vi "ProgramFreqBulk.vi"(8 "error in (no error)":errorcluster, 9 "auto start":bool=TRUE, 11 "RUS settings":T1={"NI-DAQ lockin settings"={"Samples per sine wave"=0, "Sine waves per freq step"=0, "Output Representation"=enum."Real/Imaginary", "Low-pass filter"=enum."Butterworth", "Ranges and couplings "=[]}, "Fast swep settings"={"Update rate (Hz)"=250.0, "Start F, Hz"=200000.0, "Stop F"=1700000.0, "Number of points"=30000, "Amplitude"=2.1, "Init&amplitude"=TRUE, "IF"=1000.0, "Time constant"=0.1}, "Pre-sweep delay, s"=0.0, "Lockin mode"=enum."NI-DAQ", "SR Lockin"="GPIB0::10::INSTR", "DAQmx Device"="Dev3", "Clock Multiplier"=64, "Fast Sweep Data Out"={"DO clock task"="", "DO task"="", "Update clock task"="", "DAQ lockin task"="", "Pre-sweep counter task"=""}, "Lockin Range, V"=0.0, "F Array"=[], "Freq. update clock terminal"="", "DO Clock Rate (Hz)"=5000000.0, "ADC clock terminal"="/PFI4", "Pre-sweep counter terminal"="", "Samples per read"=10, "DO clock terminal"="", "Pre-sweep points"=0, "F points per write"=1000, "Total sweep time, s"=0.0, "Initial SYNTH phase"=0.0, "Record IF"=FALSE, "Save data settings"={"Save data"=TRUE, "Data Root Path"=path "", "File Prefix"="", "File Format"=enum."ASCII", "Save column names"=TRUE, "File Comments"="<Description of the current file>", "User/Prj"="<User Name/Project Description>"}, "Data file path"=path "", "New data user event"=refnum, "Stop user event"=refnum, "Number of channels"=1, "Auto-phase"=FALSE, "RP Transeiver"=refnum} {"Lockin Range, V" format="%#_6e"; "Fast swep settings"."IF" format="%#_6p"; "Fast swep settings"."Amplitude" min=0.0 max=2.5; "Fast swep settings"."Number of points" format="%.0p"; "Fast swep settings"."Stop F" format="%#_6p"; "Fast swep settings"."Start F, Hz" format="%#_6p"; "Fast swep settings"."Update rate (Hz)" format="%0.2f"; "NI-DAQ lockin settings"."Ranges and couplings"."Coupling" items=["default"=-1, "RSE"=10083, "NRSE"=10078, "Differential"=10106, "Pseudodifferential"=12529]}) -> (0 "error out":errorcluster, 2 "SpaceAvail":u32, 3 "RUS settings out":T1={"NI-DAQ lockin settings"={"Samples per sine wave"=0, "Sine waves per freq step"=0, "Output Representation"=enum."Real/Imaginary", "Low-pass filter"=enum."Butterworth", "Ranges and couplings "=[]}, "Fast swep settings"={"Update rate (Hz)"=250.0, "Start F, Hz"=200000.0, "Stop F"=1700000.0, "Number of points"=30000, "Amplitude"=2.1, "Init&amplitude"=TRUE, "IF"=1000.0, "Time constant"=0.1}, "Pre-sweep delay, s"=0.0, "Lockin mode"=enum."NI-DAQ", "SR Lockin"="GPIB0::10::INSTR", "DAQmx Device"="Dev3", "Clock Multiplier"=64, "Fast Sweep Data Out"={"DO clock task"="", "DO task"="", "Update clock task"="", "DAQ lockin task"="", "Pre-sweep counter task"=""}, "Lockin Range, V"=0.0, "F Array"=[], "Freq. update clock terminal"="", "DO Clock Rate (Hz)"=5000000.0, "ADC clock terminal"="/PFI4", "Pre-sweep counter terminal"="", "Samples per read"=10, "DO clock terminal"="", "Pre-sweep points"=0, "F points per write"=1000, "Total sweep time, s"=0.0, "Initial SYNTH phase"=0.0, "Record IF"=FALSE, "Save data settings"={"Save data"=TRUE, "Data Root Path"=path "", "File Prefix"="", "File Format"=enum."ASCII", "Save column names"=TRUE, "File Comments"="<Description of the current file>", "User/Prj"="<User Name/Project Description>"}, "Data file path"=path "", "New data user event"=refnum, "Stop user event"=refnum, "Number of channels"=1, "Auto-phase"=FALSE, "RP Transeiver"=refnum} {"Lockin Range, V" format="%#_6e"; "Fast swep settings"."IF" format="%#_6p"; "Fast swep settings"."Amplitude" min=0.0 max=2.5; "Fast swep settings"."Number of points" format="%.0p"; "Fast swep settings"."Stop F" format="%#_6p"; "Fast swep settings"."Start F, Hz" format="%#_6p"; "Fast swep settings"."Update rate (Hz)" format="%0.2f"; "NI-DAQ lockin settings"."Ranges and couplings"."Coupling" items=["default"=-1, "RSE"=10083, "NRSE"=10078, "Differential"=10106, "Pseudodifferential"=12529]}, 4 "DO array  making time":u32, 6 "DO write time":u32)   [LabVIEW 2015]
uses:
  RUS/Controls/RUS settings.ctl
  NHMFL_Core/Libraries/Red Pitaya/RP Core/RP Transceiver/RP Transceiver.lvclass
  RUS/Controls/RUS NI-DAQ Lockin Settings.ctl
  RUS/Controls/Sweep settings.ctl
  RUS/Controls/Lockin mode.ctl
  NHMFL_Core/Libraries/File/Controls/Save data settings.ctl
  NHMFL_Core/Libraries/File/Controls/File formats.ctl
  <vilib>/DAQmx/write.llb/DAQmx Write (Digital 1D U8 1Chan NSamp).vi
  <vilib>/DAQmx/miscellaneous.llb/DAQmx Fill In Error Info.vi
  <resource>/objmgr/daqmx.rc
panel:
  in  "auto start 2":bool=TRUE
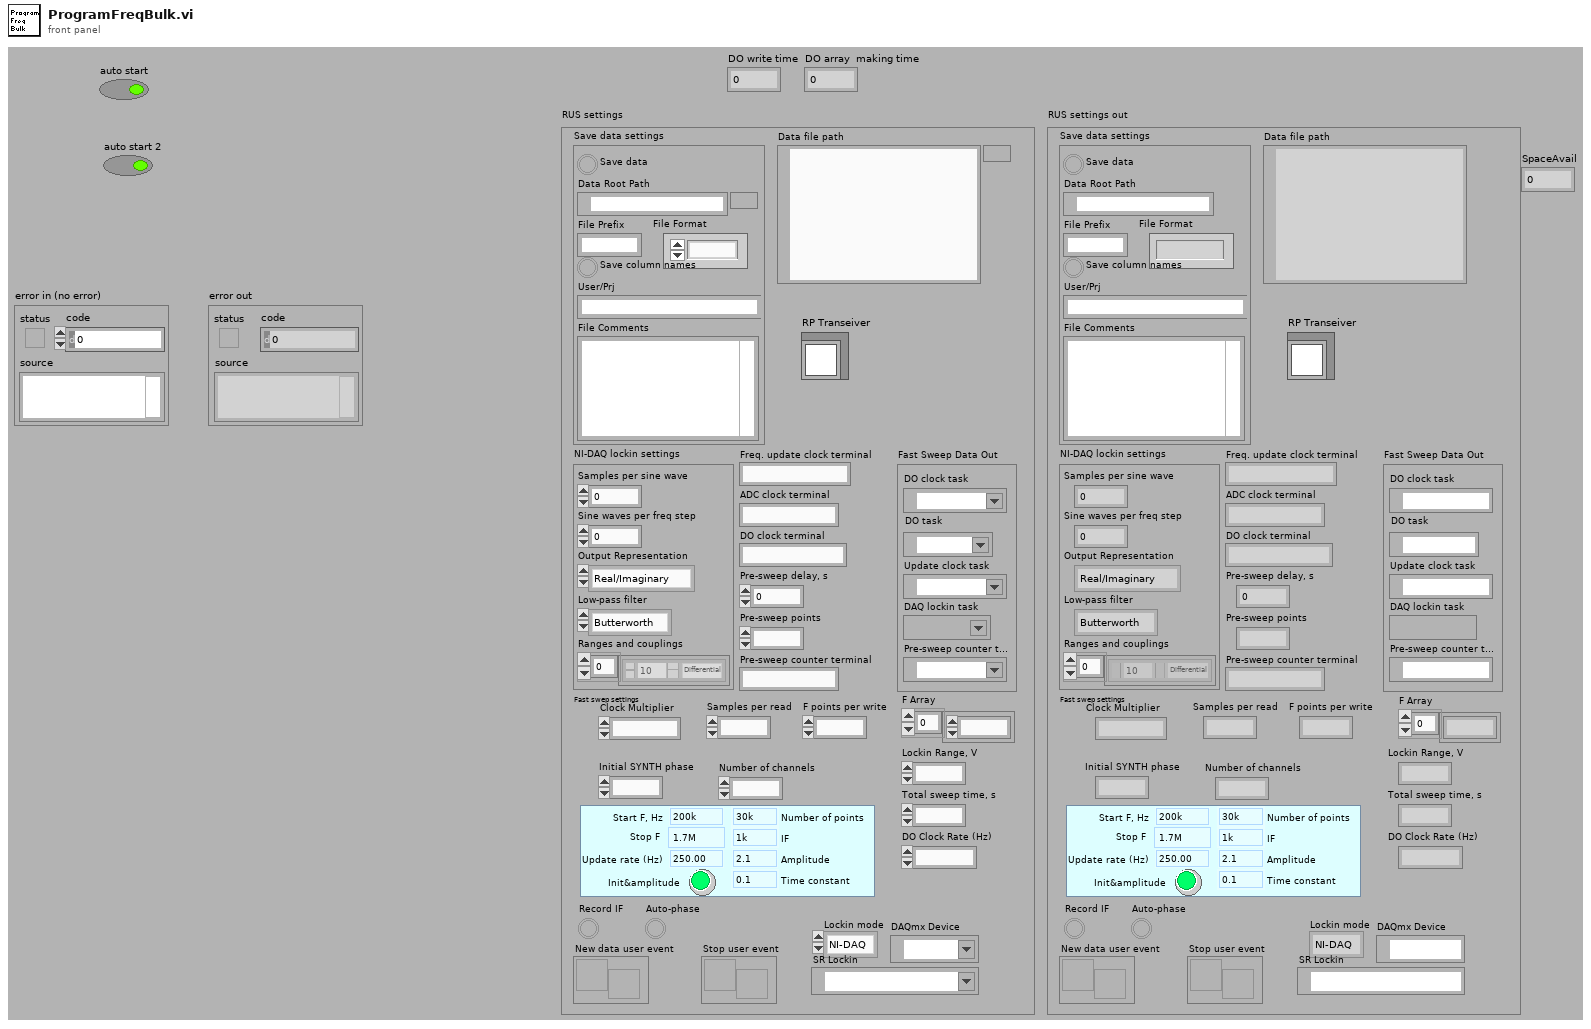
[diagram p1: front panel]
types:
  T1 = typedef "RUS settings.ctl" = cluster{"NI-DAQ lockin settings":T2, "Fast swep settings":T3, "Pre-sweep delay, s":dbl, "Lockin mode":T4, "SR Lockin":refnum<visa-resource-name>, "DAQmx Device":tag, "Clock Multiplier":i32, "Fast Sweep Data Out":cluster{"DO clock task":refnum<k21>, "DO task":refnum<k21>, "Update clock task":refnum<k21>, "DAQ lockin task":refnum<k21>, "Pre-sweep counter task":refnum<k21>}, "Lockin Range, V":sgl, "F Array":dbl[], "Freq. update clock terminal":string, "DO Clock Rate (Hz)":dbl, "ADC clock terminal":string, "Pre-sweep counter terminal":string, "Samples per read":i32, "DO clock terminal":string, "Pre-sweep points":i32, "F points per write":i32, "Total sweep time, s":dbl, "Initial SYNTH phase":dbl, "Record IF":bool, "Save data settings":T5, "Data file path":path, "New data user event":refnum<user-event>, "Stop user event":refnum<user-event>, "Number of channels":i32, "Auto-phase":bool, "RP Transeiver":refnum<class "RP Transceiver.lvclass">}
  T2 = typedef "RUS NI-DAQ Lockin Settings.ctl" = cluster{"Samples per sine wave":i32, "Sine waves per freq step":i32, "Output Representation":enum16{"Real/Imaginary", "Polar"}, "Low-pass filter":enum16{"No filtering", "Butterworth", "Bessel"}, "Ranges and couplings ":cluster{"Range":dbl, "Coupling":i32}[]}
  T3 = typedef "Sweep settings.ctl" = cluster{"Update rate (Hz)":dbl, "Start F, Hz":dbl, "Stop F":dbl, "Number of points":i32, "Amplitude":dbl, "Init&amplitude":bool, "IF":dbl, "Time constant":dbl}
  T4 = typedef "Lockin mode.ctl" = enum16{"SRS", "NI-DAQ", "Pitaya"}
  T5 = typedef "Save data settings.ctl" = cluster{"Save data":bool, "Data Root Path":path, "File Prefix":string, "File Format":T6, "Save column names":bool, "File Comments":string, "User/Prj":string}
  T6 = typedef "File formats.ctl" = enum16{"TDMS", "ASCII", "BINARY"}
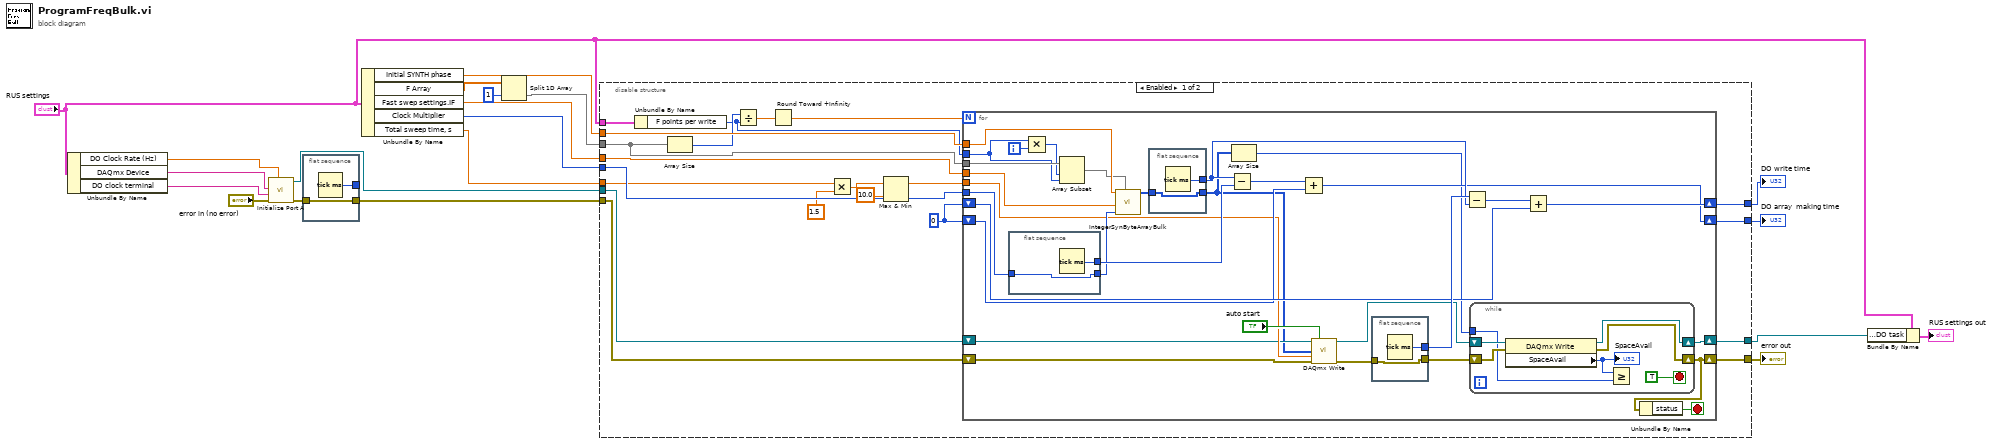
[diagram p0: block diagram]
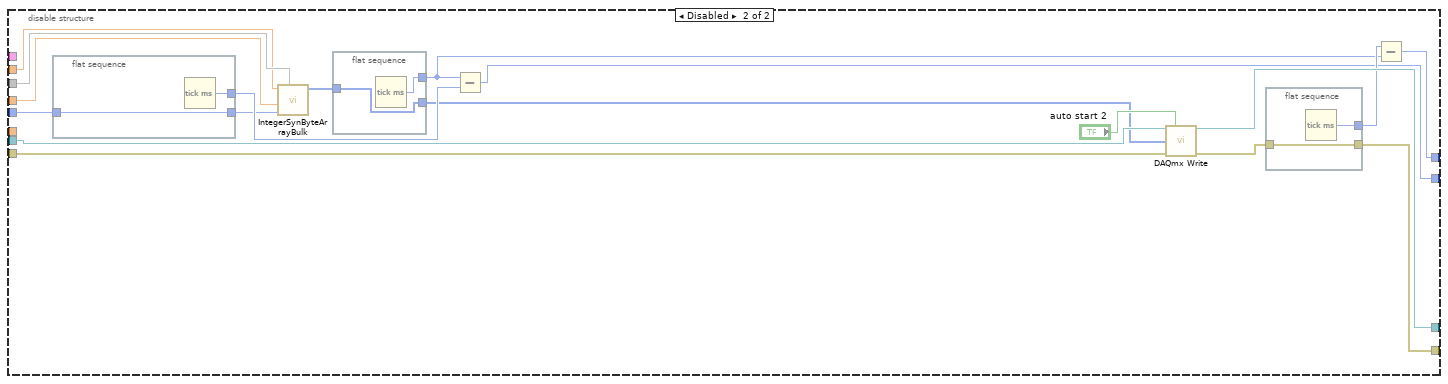
[diagram p2: hidden frame]
diagram:
  n1 = Unbundle By Name("RUS settings") -> ("DO Clock Rate (Hz)"=w14:dbl, "DAQmx Device"=w15:tag, "DO clock terminal"=w16:string)
  n2 = call "Initialize Port A.VI"("DO Clock Rate (Hz)"=w14, "error in (no error)"="error in (no error)", "Clock source"=w16, "DAQmx Device Name"=w15) -> ("error out"=w11:errorcluster, "task out"=w19:refnum<k21>)  [unwired: 3 in, 3 out]
  n3 = flat-sequence {
    tunnel: [w22] -> w10
    tunnel: w11 -> [w22]
    tunnel: [w21] -> _
    frame #0 {
      n4 = Tick Count (ms)() -> (millisecond timer value=w21:u32)
    }
  }
  n5 = Unbundle By Name("RUS settings") -> ("Initial SYNTH phase"=w3:dbl, "F Array"=w7:dbl[], "Fast swep settings.IF"=w6:dbl, "Clock Multiplier"=w13:i32, "Total sweep time, s"=w4:dbl)
  n6 = Split 1D Array(array=w7, index=1) -> (second subarray=w2:dbl[])  [unwired: 1 out]
  n7 = disable-structure shown="Enabled" {
    disable-tunnel: w19 -> [w25 w104]
    disable-tunnel: [w43 w103] -> w17
    disable-tunnel: w13 -> [w42 w102]
    disable-tunnel: [w41 w100] -> w12
    disable-tunnel: w10 -> [w24 w99]
    disable-tunnel: [w40 w97] -> w9
    disable-tunnel: [w39 w95] -> w8
    disable-tunnel: w2 -> [w37 w94]
    disable-tunnel: w3 -> [w38 w93]
    disable-tunnel: w6 -> [w33 w92]
    disable-tunnel: "RUS settings" -> [w27 _]
    disable-tunnel: w4 -> [w23 _]
    frame Enabled {
      w34 = u32 0
      n8 = Unbundle By Name(w27) -> ("F points per write"=w26:i32)
      n9 = Array Size(array=w37) -> (size(s)=w32:i32)
      n10 = Divide(x=w32, y=w26) -> (x/y=w36:dbl)
      n11 = Round Toward +Infinity(x=w36) -> (ceil(x): smallest int >= x=w35:dbl)
      n12 = Multiply(x=w23, y=1.5) -> (x*y=w29:dbl)
      n13 = Max & Min(x=w29, y=10.0) -> (max(x,y)=w30:dbl)  [unwired: 1 out]
      n14 = for {
        N: w35 -> [_]
        tunnel: w42 -> [w73]
        tunnel: w37 -> [w62]
        tunnel: w38 -> [w67]
        tunnel: w33 -> [w66]
        shift-right: [w45] -> w41
        shift-left: w24 -> [w52]
        shift-right: [w48] -> w43
        shift-left: w25 -> [w49]
        shift-right: [w60] -> w40
        shift-left: w34 -> [w59]
        shift-right: [w58] -> w39
        shift-left: w34 -> [w57]
        tunnel: w26 -> [w55]
        tunnel: w30 -> [w53]
        i -> [w56]
        stop <- w44 stop-if-true
        n15 = flat-sequence {
          tunnel: [w87] -> w65
          tunnel: w73 -> [w87]
          tunnel: [w86] -> w69
          frame #0 {
            n16 = Tick Count (ms)() -> (millisecond timer value=w86:u32)
          }
        }
        n17 = Multiply(x=w55, y=w56) -> (x*y=w54:i32)
        n18 = Array Subset(array=w62, index=w54, length=w55) -> (w61:dbl[])
        n19 = call "IntegerSynByteArrayBulk.vi"("Input  F1 array"=w61, "Clock multiplier"=w65, "Local Oscillator (IF,f2)"=w66, "Phase (degrees)"=w67) -> ("output array"=w64:u8[])  [unwired: 7 in]
        n20 = flat-sequence {
          tunnel: [w83] -> w47
          tunnel: w64 -> [w83]
          tunnel: [w82] -> w63
          frame #0 {
            n21 = Tick Count (ms)() -> (millisecond timer value=w82:u32)
          }
        }
        n22 = Subtract(x=w63, y=w69) -> (x-y=w68:u32)
        n23 = Array Size(array=w47) -> (size(s)=w46:i32)
        n24 = Add(x=w68, y=w57) -> (x+y=w58:u32)
        n25 = call-poly <vilib>:"DAQmx Write.vi"("task/channels in"=w49, "auto start"="auto start", "data"=w47, "timeout"=w53, "error in"=w52) -> ("task out"=w50:refnum<k21>, "error out"=w72:errorcluster)  [unwired: 9 out]
        n26 = flat-sequence {
          tunnel: [w85] -> w51
          tunnel: w72 -> [w85]
          tunnel: [w84] -> w71
          frame #0 {
            n27 = Tick Count (ms)() -> (millisecond timer value=w84:u32)
          }
        }
        n28 = Subtract(x=w71, y=w63) -> (x-y=w70:u32)
        n29 = while {
          shift-right: [w79] -> w48
          shift-left: w50 -> [w80]
          shift-right: [w78] -> w45
          shift-left: w51 -> [w81]
          tunnel: w46 -> [w76]
          stop <- TRUE stop-if-true
          n30 = property class="DAQmx Write"(reference=w80, error in=w81) -> (reference out=w79:refnum<k21>, error out=w78:errorcluster, "SpaceAvail"=w77:u32)
          "SpaceAvail" <- w77
          n31 = Greater Or Equal?(x=w77, y=w76) -> ()  [unwired: 1 out]
        }
        n32 = Add(x=w70, y=w59) -> (x+y=w60:u32)
        n33 = Unbundle By Name(w45) -> ("status"=w44:bool)
      }
    }
    frame Disabled {
      n34 = flat-sequence {
        tunnel: [w111] -> w91
        tunnel: w102 -> [w111]
        tunnel: [w110] -> w96
        frame #0 {
          n35 = Tick Count (ms)() -> (millisecond timer value=w110:u32)
        }
      }
      n36 = call "IntegerSynByteArrayBulk.vi"("Input  F1 array"=w94, "Clock multiplier"=w91, "Local Oscillator (IF,f2)"=w92, "Phase (degrees)"=w93) -> ("output array"=w90:u8[])  [unwired: 7 in]
      n37 = flat-sequence {
        tunnel: [w107] -> w89
        tunnel: w90 -> [w107]
        tunnel: [w106] -> w88
        frame #0 {
          n38 = Tick Count (ms)() -> (millisecond timer value=w106:u32)
        }
      }
      n39 = Subtract(x=w88, y=w96) -> (x-y=w95:u32)
      n40 = call-poly <vilib>:"DAQmx Write.vi"("task/channels in"=w104, "auto start"="auto start 2", "data"=w89, "error in"=w99) -> ("task out"=w103:refnum<k21>, "error out"=w101:errorcluster)  [unwired: 10 out]
      n41 = flat-sequence {
        tunnel: [w109] -> w100
        tunnel: w101 -> [w109]
        tunnel: [w108] -> w98
        frame #0 {
          n42 = Tick Count (ms)() -> (millisecond timer value=w108:u32)
        }
      }
      n43 = Subtract(x=w98, y=w88) -> (x-y=w97:u32)
    }
  }
  "error out" <- w12
  "DO write time" <- w9
  "DO array  making time" <- w8
  n44 = Bundle By Name(cluster="RUS settings", "Fast Sweep Data Out.DO task"=w17) -> (→"RUS settings out":T1)
